vi "Load Supported Music Libraries.vi"(8 "error in (no error)":errorcluster, 11 "Supported Music Libraries Paths":path[](array[path])) -> (0 "error out":errorcluster, 3 "Supported Files":refnum<class "MusicFile.lvclass">[](array[class]))   [LabVIEW 2015, in "MusicFile.lvclass"]
uses:
  MusicFile.lvclass
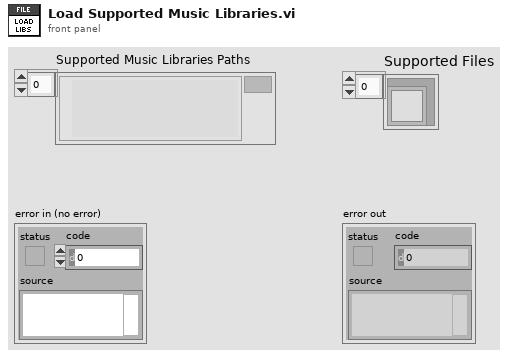
[diagram p1: front panel]
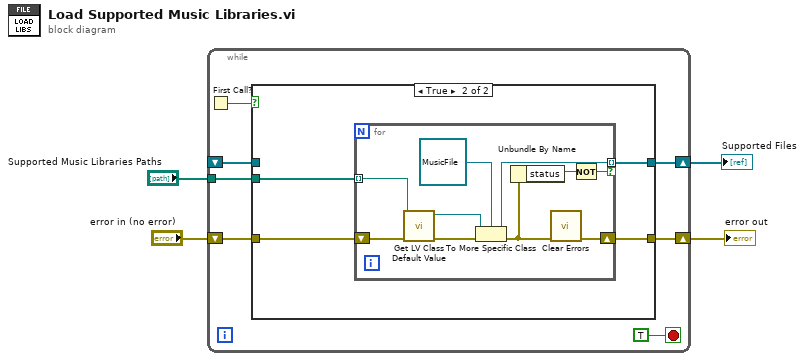
[diagram p0: block diagram]
diagram:
  n1 = while {
    shift-right: [w10] -> w3
    shift-left: "error in (no error)" -> [w11]
    shift-right: [w7] -> w1
    shift-left: _ -> [w6]
    tunnel: "Supported Music Libraries Paths" -> [w5]
    stop <- TRUE stop-if-true
    n2 = First Call?() -> (First Call?: T/F=w9:bool)
    n3 = case shown="True" w9 {
      tunnel: [w13 w17] -> w10
      tunnel: w11 -> [w13 w15]
      tunnel: [w12 w16] -> w7
      tunnel: w6 -> [w12 _]
      tunnel: w5 -> [_ w14]
      frame False {
      }
      frame True {
        n4 = for {
          shift-right: [w22] -> w17
          shift-left: w15 -> [w27]
          tunnel: w14 -> [w26] mode=indexing
          tunnel: [w23] -> w16 mode=indexing if=w20
          n5 = call <vilib>:"Get LV Class Default Value.vi"("error in (no error)"=w27, "class path"=w26) -> ("error out"=w25:errorcluster, "object"=w24:refnum<class>)  [unwired: 8 in]
          n6 = To More Specific Class(target class=refnum<class "MusicFile.lvclass"> refnum ("MusicFile.lvclass"), reference=w24, error in=w25) -> (specific class reference=w23:refnum<class "MusicFile.lvclass">, error out=w21:errorcluster)
          n7 = Unbundle By Name(w21) -> ("status"=w19:bool)
          n8 = call <vilib>:"Clear Errors.vi"("error in (no error)"=w21) -> ("error out"=w22:errorcluster)  [unwired: 5 in, 1 out]
          n9 = Not(x=w19) -> (.not. x?=w20:bool)
        }
      }
    }
  }
  "error out" <- w3
  "Supported Files" <- w1
